vi "Apply Default.vi"(11 "Type in":refnum<class "Type.lvclass">) -> (3 "Type out":refnum<class "Type.lvclass">)   [LabVIEW 2020, in "Conditum.lvlib" / "Columns.lvlib" / "Type.lvclass"]
uses:
  Type.lvclass
  Type.lvclass/Type.ctl
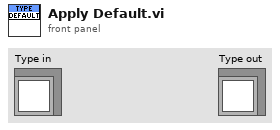
[diagram p1: front panel]
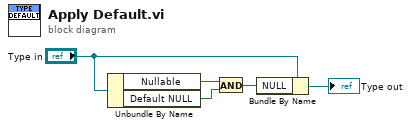
[diagram p0: block diagram]
diagram:
  n1 = Unbundle By Name("Type in") -> ("Nullable"=w5:bool, "Default NULL"=w4:bool)
  n2 = And(x=w5, y=w4) -> (x .and. y?=w2:bool)
  n3 = Bundle By Name(cluster="Type in", "NULL"=w2) -> (→"Type out":refnum<class "Type.lvclass">)
